vi "ep_AC Coupling.vi"(0 "phase voltage waveforms in":waveform(dbl)[](array[waveform]), 5 "current waveforms in":waveform(dbl)[](array[waveform]), 11 "error in (no error)":errorcluster) -> (4 "phase voltage waveforms out":waveform(dbl)[](array[waveform]), 6 "current waveforms out":waveform(dbl)[](array[waveform]), 15 "error out":errorcluster)   [LabVIEW 2014, in "NI_EP_Motor Monitoring.lvlib"]
uses:
  <vilib>/addons/Electrical Power/Motor Monitoring/NI_EP_Motor Monitoring.lvlib
  <vilib>/Analysis/NI_AALPro.lvlib
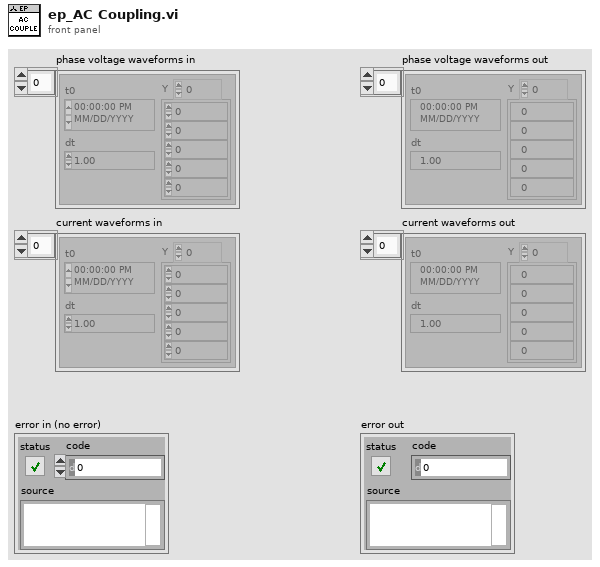
[diagram p1: front panel]
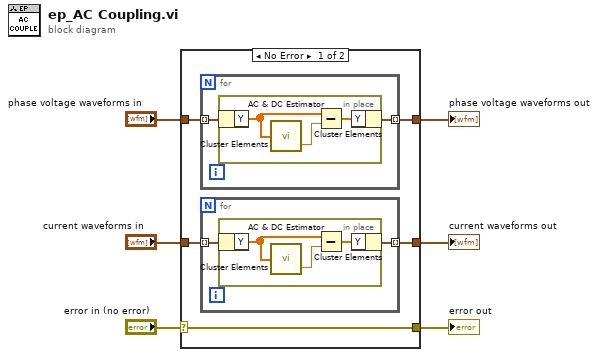
[diagram p0: block diagram]
diagram:
  n1 = case shown="No Error" "error in (no error)" {
    selector: "error in (no error)" -> [w9 w22]
    tunnel: [w11 _] -> w6
    tunnel: "phase voltage waveforms in" -> [w10 _]
    tunnel: "current waveforms in" -> [w8 _]
    tunnel: [w7 _] -> w3
    tunnel: [w9 w22] -> w1
    frame No Error {
      n2 = for {
        tunnel: w10 -> [w18] mode=indexing
        tunnel: [w17] -> w11 mode=indexing
        n3 = in-place {
          n4 = in-place-cluster #1(w18) -> ("Y"=w21:dbl[])
          n5 = call <vilib>:"AC & DC Estimator.vi"("Signal (V)"=w21) -> ("DC estimate (V)"=w19:dbl)  [unwired: 1 out]
          n6 = Subtract(x=w21, y=w19) -> (x-y=w20:dbl[])
          n7 = in-place-cluster #1("Y"=w20) -> (w17:waveform(dbl))
        }
      }
      n8 = for {
        tunnel: w8 -> [w13] mode=indexing
        tunnel: [w12] -> w7 mode=indexing
        n9 = in-place {
          n10 = in-place-cluster #2(w13) -> ("Y"=w16:dbl[])
          n11 = call <vilib>:"AC & DC Estimator.vi"("Signal (V)"=w16) -> ("DC estimate (V)"=w14:dbl)  [unwired: 1 out]
          n12 = Subtract(x=w16, y=w14) -> (x-y=w15:dbl[])
          n13 = in-place-cluster #2("Y"=w15) -> (w12:waveform(dbl))
        }
      }
    }
    frame Error {
    }
  }
  "error out" <- w1
  "current waveforms out" <- w3
  "phase voltage waveforms out" <- w6
